vi "OSICS_Set_Enable_Disable.vi"(7 "OSICS slot":i32=1 min=1 max=8 step=1, 8 "error in":errorcluster, 10 "Laser State (False:DISABLED)":bool, 11 "VISA IN":refnum<visa-resource-name>) -> (0 "error out":errorcluster, 3 "VISA OUT":refnum<visa-resource-name>, 5 "ERR":i32)   [LabVIEW 2014, in "OSICS_LIB.lvlib"]
doc: "This Vi enables/disables the optical output of OSICS Modules."
uses:
  OSICS_LIB.lvlib
panel:
  # "BASIC Function to Enable/Disable OSICS modules"
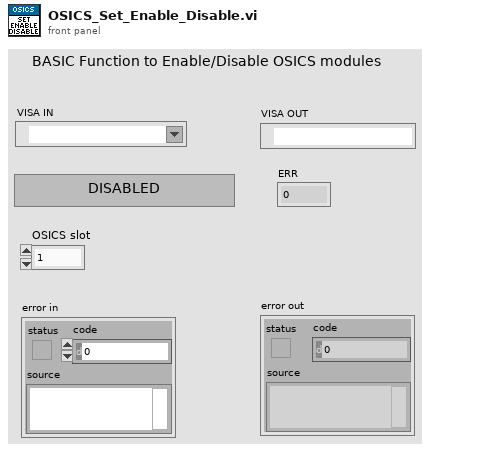
[diagram p1: front panel]
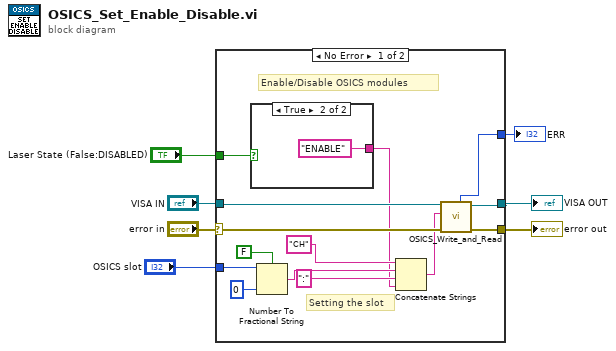
[diagram p0: block diagram]
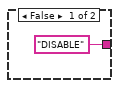
[diagram p2: hidden frame]
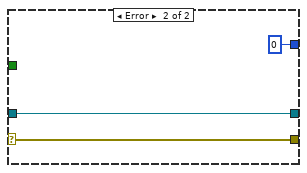
[diagram p3: hidden frame]
diagram:
  n1 = case shown="No Error" "error in" {
    selector: "error in" -> [w18 w25]
    tunnel: "VISA IN" -> [w19 w26]
    tunnel: [w21 w26] -> w6
    tunnel: [w20 w25] -> w5
    tunnel: "Laser State (False:DISABLED)" -> [w17 _]
    tunnel: [w8 0 ("ERR")] -> w2
    tunnel: "OSICS slot" -> [w15 _]
    frame No Error {
      # "Setting the slot"
      # "Enable/Disable OSICS modules"
      n2 = case shown="True" w17 {
        tunnel: ["DISABLE" "ENABLE"] -> w10
        frame False {
        }
        frame True {
        }
      }
      n3 = Number To Fractional String(use system decimal point (T)=FALSE, number=w15, precision (6)=i16 0) -> (F-format string=w13:string)  [unwired: 1 in]
      n4 = Concatenate Strings("CH" ("string"), w13, ":" ("string"), w10) -> (w11:string)
      n5 = call "OSICS_Write_and_Read.vi"("error in (no error)"=w18, "String to Send"=w11, "VISA IN"=w19) -> ("error out"=w20:errorcluster, "VISA OUT"=w21:refnum<visa-resource-name>, "ERR"=w8:i32)  [unwired: 5 in, 1 out]
    }
    frame Error {
    }
  }
  "error out" <- w5
  "VISA OUT" <- w6
  "ERR" <- w2
